vi "pumpControl.vi"(0 "OFF":bool, 8 "pump number":i32=1, 10 "vol":dbl caption="vol_p1" format="%.1f") -> ()   [LabVIEW 2021]
uses:
  <vilib>/Utility/error.llb/DialogType.ctl
  <vilib>/DAQmx/write.llb/DAQmx Write (Digital Bool 1Line 1Point).vi
  <vilib>/DAQmx/write.llb/DAQmx Write (Analog DBL 1Chan 1Samp).vi
  globalVariables.vi
  <vilib>/DAQmx/create/channels.llb/DAQmx Create Channel (DO-Digital Output).vi
  <vilib>/DAQmx/miscellaneous.llb/DAQmx Fill In Error Info.vi
  <vilib>/DAQmx/create/channels.llb/DAQmx Create Channel (AO-Voltage-Basic).vi
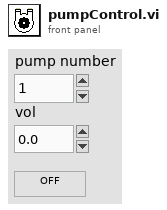
[diagram p1: front panel]
types:
  T1 = typedef "DialogType.ctl" = u16
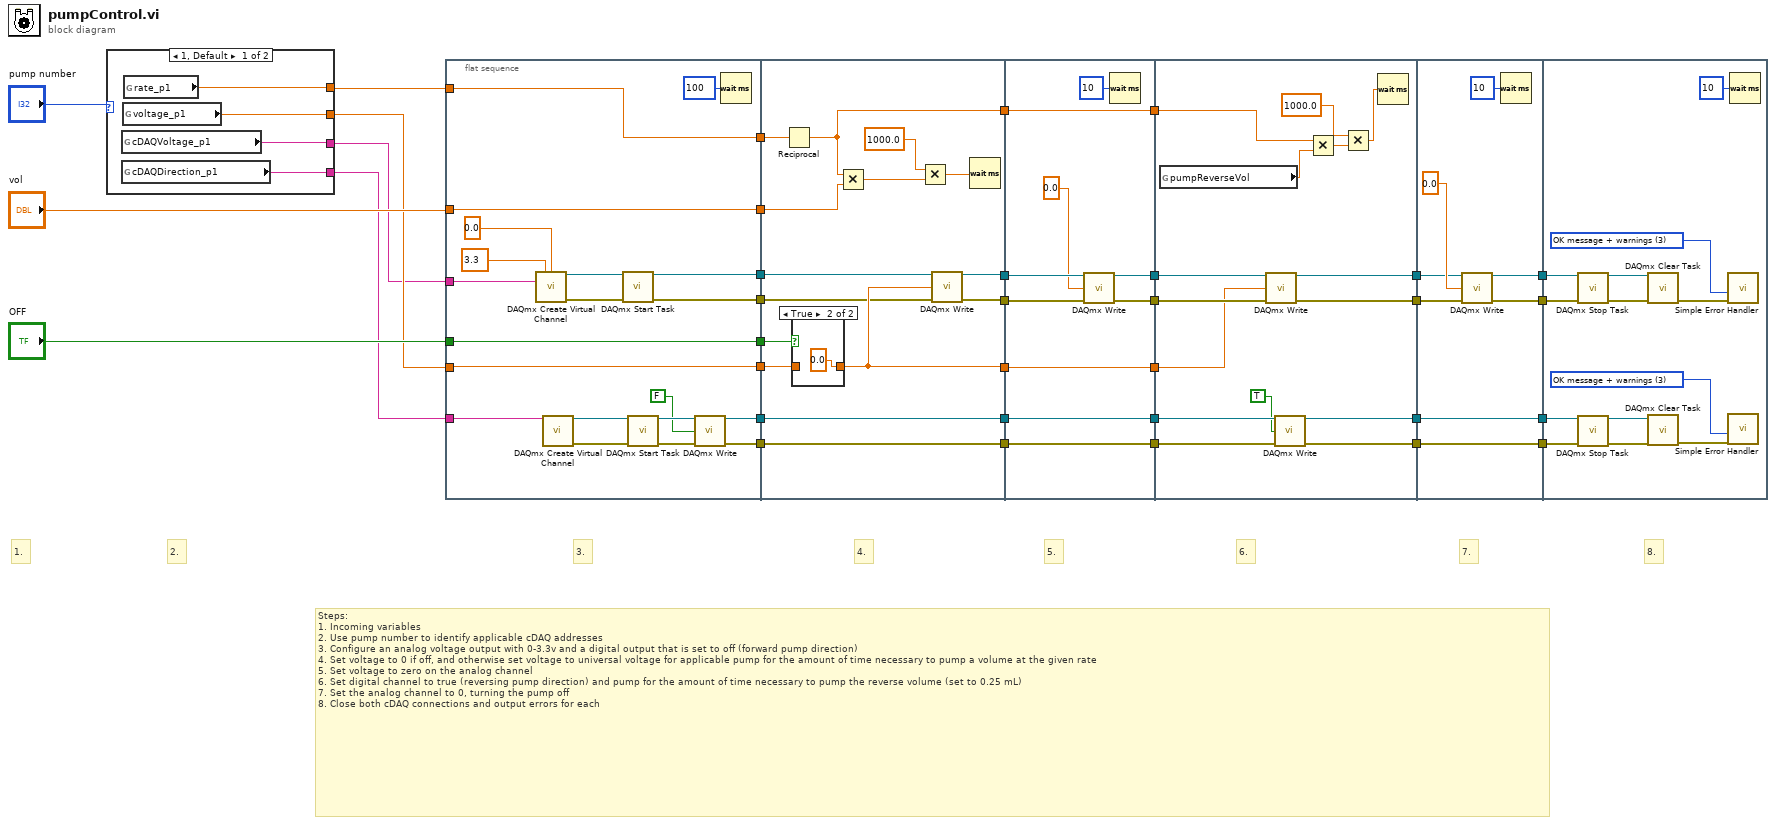
[diagram p0: block diagram]
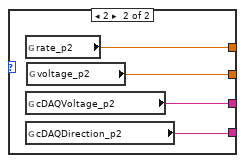
[diagram p2: hidden frame]
diagram:
  # "Steps:\n1. Incoming variables\n2. Use pump number to identify applicable cDAQ addresses\n3. Configure an analog voltage output with 0-3.3v and a digital output that is set to off (forward pump direction)\n4. Set voltage to 0 if off, and otherwise set voltage to universal voltage for applicable pump for the amount of time necessary to pump a volume at the given rate\n5. Set voltage to zero on the analog channel\n6. Set digital channel to true (reversing pump direction) and pump for the amount of time necessary to pump the reverse volume (set to 0.25 mL)\n7. Set the analog channel to 0, turning the pump off\n8. Close both cDAQ connections and output errors for each"
  # "8."
  # "7."
  # "6."
  # "5."
  # "4."
  # "3."
  # "2."
  # "1."
  n1 = case shown="1, Default" "pump number" {
    tunnel: [w39 w43] -> w12
    tunnel: [w38 w42] -> w11
    tunnel: [w37 w41] -> w10
    tunnel: [w36 w40] -> w9
    frame 1, Default {
      n2 = global read "globalVariables.vi" "cDAQVoltage_p1"() -> (w37:tag)
      n3 = global read "globalVariables.vi" "cDAQDirection_p1"() -> (w36:tag)
      n4 = global read "globalVariables.vi" "voltage_p1"() -> (w38:dbl)
      n5 = global read "globalVariables.vi" "rate_p1"() -> (w39:dbl)
    }
    frame 2 {
      n6 = global read "globalVariables.vi" "rate_p2"() -> (w43:dbl)
      n7 = global read "globalVariables.vi" "cDAQVoltage_p2"() -> (w41:tag)
      n8 = global read "globalVariables.vi" "cDAQDirection_p2"() -> (w40:tag)
      n9 = global read "globalVariables.vi" "voltage_p2"() -> (w42:dbl)
    }
  }
  n10 = flat-sequence {
    tunnel: w9 -> [w59]
    tunnel: w10 -> [w46]
    tunnel: w11 -> [w60]
    tunnel: w12 -> [w61]
    tunnel: "vol" -> [w62]
    tunnel: "OFF" -> [w63]
    tunnel: [w63] -> w8
    tunnel: [w62] -> w7
    tunnel: [w61] -> w6
    tunnel: [w60] -> w5
    tunnel: [w53] -> w4
    tunnel: [w52] -> w3
    tunnel: [w45] -> w2
    tunnel: [w44] -> w1
    tunnel: [w74] -> w33
    tunnel: [w73] -> w32
    tunnel: [w71] -> w24
    tunnel: [w67] -> w20
    tunnel: [w66] -> w16
    tunnel: [w70] -> w14
    tunnel: w8 -> [w78]
    tunnel: w7 -> [w75]
    tunnel: w6 -> [w69]
    tunnel: w5 -> [w68]
    tunnel: w4 -> [w67]
    tunnel: w3 -> [w66]
    tunnel: w2 -> [w65]
    tunnel: w1 -> [w64]
    tunnel: w33 -> [w90]
    tunnel: w32 -> [w88]
    tunnel: [w87] -> w31
    tunnel: [w86] -> w30
    tunnel: [w84] -> w25
    tunnel: w24 -> [w84]
    tunnel: [w83] -> w21
    tunnel: w20 -> [w83]
    tunnel: [w82] -> w17
    tunnel: w16 -> [w82]
    tunnel: [w81] -> w15
    tunnel: w14 -> [w81]
    tunnel: w31 -> [w103]
    tunnel: w30 -> [w102]
    tunnel: [w104] -> w29
    tunnel: [w105] -> w26
    tunnel: w25 -> [w98]
    tunnel: [w96] -> w22
    tunnel: w21 -> [w97]
    tunnel: [w94] -> w18
    tunnel: w17 -> [w95]
    tunnel: w15 -> [w92]
    tunnel: w29 -> [w109]
    tunnel: [w108] -> w28
    tunnel: [w110] -> w27
    tunnel: w26 -> [w111]
    tunnel: [w107] -> w23
    tunnel: w22 -> [w107]
    tunnel: [w106] -> w19
    tunnel: w18 -> [w106]
    tunnel: w28 -> [w124]
    tunnel: w27 -> [w125]
    tunnel: w23 -> [w119]
    tunnel: w19 -> [w118]
    frame #0 {
      n11 = call-poly <vilib>:"DAQmx Create Virtual Channel.vi"("maximum value"=3.3 ("Max Voltage"), "minimum value"=0.0 ("Min Voltage"), "physical channels"=w46) -> ("task out"=w49:refnum<k21>, "error out"=w50:errorcluster)  [unwired: 11 in]
      n12 = call-poly <vilib>:"DAQmx Create Virtual Channel.vi"("lines"=w59) -> ("task out"=w58:refnum<k21>, "error out"=w57:errorcluster)  [unwired: 13 in]
      n13 = call <vilib>:"DAQmx Start Task.vi"("task/channels in"=w49, "error in"=w50) -> ("task out"=w44:refnum<k21>, "error out"=w45:errorcluster)  [unwired: 12 in]
      n14 = call <vilib>:"DAQmx Start Task.vi"("task/channels in"=w58, "error in"=w57) -> ("task out"=w55:refnum<k21>, "error out"=w56:errorcluster)  [unwired: 12 in]
      n15 = call-poly <vilib>:"DAQmx Write.vi"("task/channels in"=w55, "data"=FALSE, "error in"=w56) -> ("task out"=w53:refnum<k21>, "error out"=w52:errorcluster)  [unwired: 10 in, 1 out]
      n16 = Wait (ms)(milliseconds to wait=u32 100) -> ()  [unwired: 1 out]
    }
    frame #1 {
      n17 = Reciprocal(x=w69) -> (1/x=w71:dbl)
      n18 = case shown="True" w78 {
        tunnel: [w79 0.0] -> w70
        tunnel: w68 -> [w79 _]
        frame False {
        }
        frame True {
        }
      }
      n19 = Multiply(x=w71, y=w75) -> (x*y=w77:dbl)
      n20 = Multiply(x=1000.0, y=w77) -> (x*y=w72:dbl)
      n21 = call-poly <vilib>:"DAQmx Write.vi"("task/channels in"=w64, "data"=w70, "error in"=w65) -> ("task out"=w74:refnum<k21>, "error out"=w73:errorcluster)  [unwired: 10 in, 1 out]
      n22 = Wait (ms)(milliseconds to wait=w72) -> ()  [unwired: 1 out]
    }
    frame #2 {
      n23 = call-poly <vilib>:"DAQmx Write.vi"("task/channels in"=w90, "data"=0.0, "error in"=w88) -> ("task out"=w87:refnum<k21>, "error out"=w86:errorcluster)  [unwired: 10 in, 1 out]
      n24 = Wait (ms)(milliseconds to wait=u32 10) -> ()  [unwired: 1 out]
    }
    frame #3 {
      n25 = global read "globalVariables.vi" "pumpReverseVol"() -> (w91:dbl)
      n26 = call-poly <vilib>:"DAQmx Write.vi"("task/channels in"=w103, "data"=w92, "error in"=w102) -> ("task out"=w105:refnum<k21>, "error out"=w104:errorcluster)  [unwired: 10 in, 1 out]
      n27 = call-poly <vilib>:"DAQmx Write.vi"("task/channels in"=w97, "data"=TRUE, "error in"=w95) -> ("task out"=w96:refnum<k21>, "error out"=w94:errorcluster)  [unwired: 10 in, 1 out]
      n28 = Multiply(x=w98, y=w91) -> (x*y=w101:dbl)
      n29 = Multiply(x=1000.0, y=w101) -> (x*y=w99:dbl)
      n30 = Wait (ms)(milliseconds to wait=w99) -> ()  [unwired: 1 out]
    }
    frame #4 {
      n31 = call-poly <vilib>:"DAQmx Write.vi"("task/channels in"=w111, "data"=0.0, "error in"=w109) -> ("task out"=w110:refnum<k21>, "error out"=w108:errorcluster)  [unwired: 10 in, 1 out]
      n32 = Wait (ms)(milliseconds to wait=u32 10) -> ()  [unwired: 1 out]
    }
    frame #5 {
      w117 = T1 3 items=["no dialog", "OK message", "continue or stop message", "OK message + warnings", "continue/stop + warnings"] ("type of dialog (OK msg:1)")
      w123 = T1 3 items=["no dialog", "OK message", "continue or stop message", "OK message + warnings", "continue/stop + warnings"] ("type of dialog (OK msg:1)")
      n33 = call <vilib>:"DAQmx Stop Task.vi"("task/channels in"=w125, "error in"=w124) -> ("task out"=w126:refnum<k21>, "error out"=w115:errorcluster)  [unwired: 12 in]
      n34 = call <vilib>:"DAQmx Stop Task.vi"("task/channels in"=w119, "error in"=w118) -> ("task out"=w121:refnum<k21>, "error out"=w122:errorcluster)  [unwired: 12 in]
      n35 = call <vilib>:"DAQmx Clear Task.vi"("task in"=w126, "error in"=w115) -> ("error out"=w114:errorcluster)  [unwired: 13 in]
      n36 = call <vilib>:"DAQmx Clear Task.vi"("task in"=w121, "error in"=w122) -> ("error out"=w120:errorcluster)  [unwired: 13 in]
      n37 = call <vilib>:"Simple Error Handler.vi"("type of dialog (OK msg:1)"=w123, "error in (no error)"=w114) -> ()  [unwired: 3 in, 5 out]
      n38 = call <vilib>:"Simple Error Handler.vi"("type of dialog (OK msg:1)"=w117, "error in (no error)"=w120) -> ()  [unwired: 3 in, 5 out]
      n39 = Wait (ms)(milliseconds to wait=u32 10) -> ()  [unwired: 1 out]
    }
  }
